vi "Range With Increment.vi"(1 "Range":cluster{"Min":dbl, "Max":dbl, "Increment":dbl}={"Min"=0.0, "Max"=0.0, "Increment"=1.0}) -> (0 "Output Array":dbl[](array[numeric]))   [LabVIEW 2010]
uses:
  <vilib>/Analysis/1siggen.llb/Ramp Pattern by Delta.vi
  <vilib>/Analysis/NI_AALBase.lvlib
panel:
  out "Samples":i32
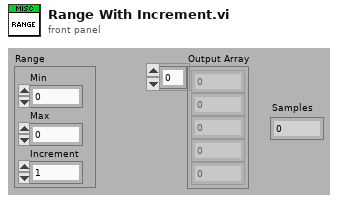
[diagram p1: front panel]
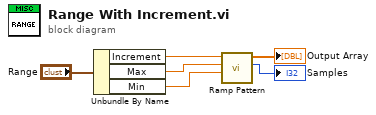
[diagram p0: block diagram]
diagram:
  n1 = Unbundle By Name("Range") -> ("Increment"=w5:dbl, "Max"=w4:dbl, "Min"=w3:dbl)
  n2 = call-poly <vilib>:"Ramp Pattern.vi"("start"=w3, "end"=w4, "delta"=w5) -> ("samples"=→"Samples":i32, "Ramp Pattern"=→"Output Array":dbl[])  [unwired: 6 in, 1 out]
